vi "final.vi"() -> ()   [LabVIEW 2022 SP3]
uses:
  <vilib>/Utility/miscctls.llb/LVRectTypeDef.ctl
panel:
  in  "3 4":bool
  out "Time/Date":string
  in  "3 3":bool
  in  "3 2":bool
  in  "3":bool
  in  "2":bool
  in  "1":bool
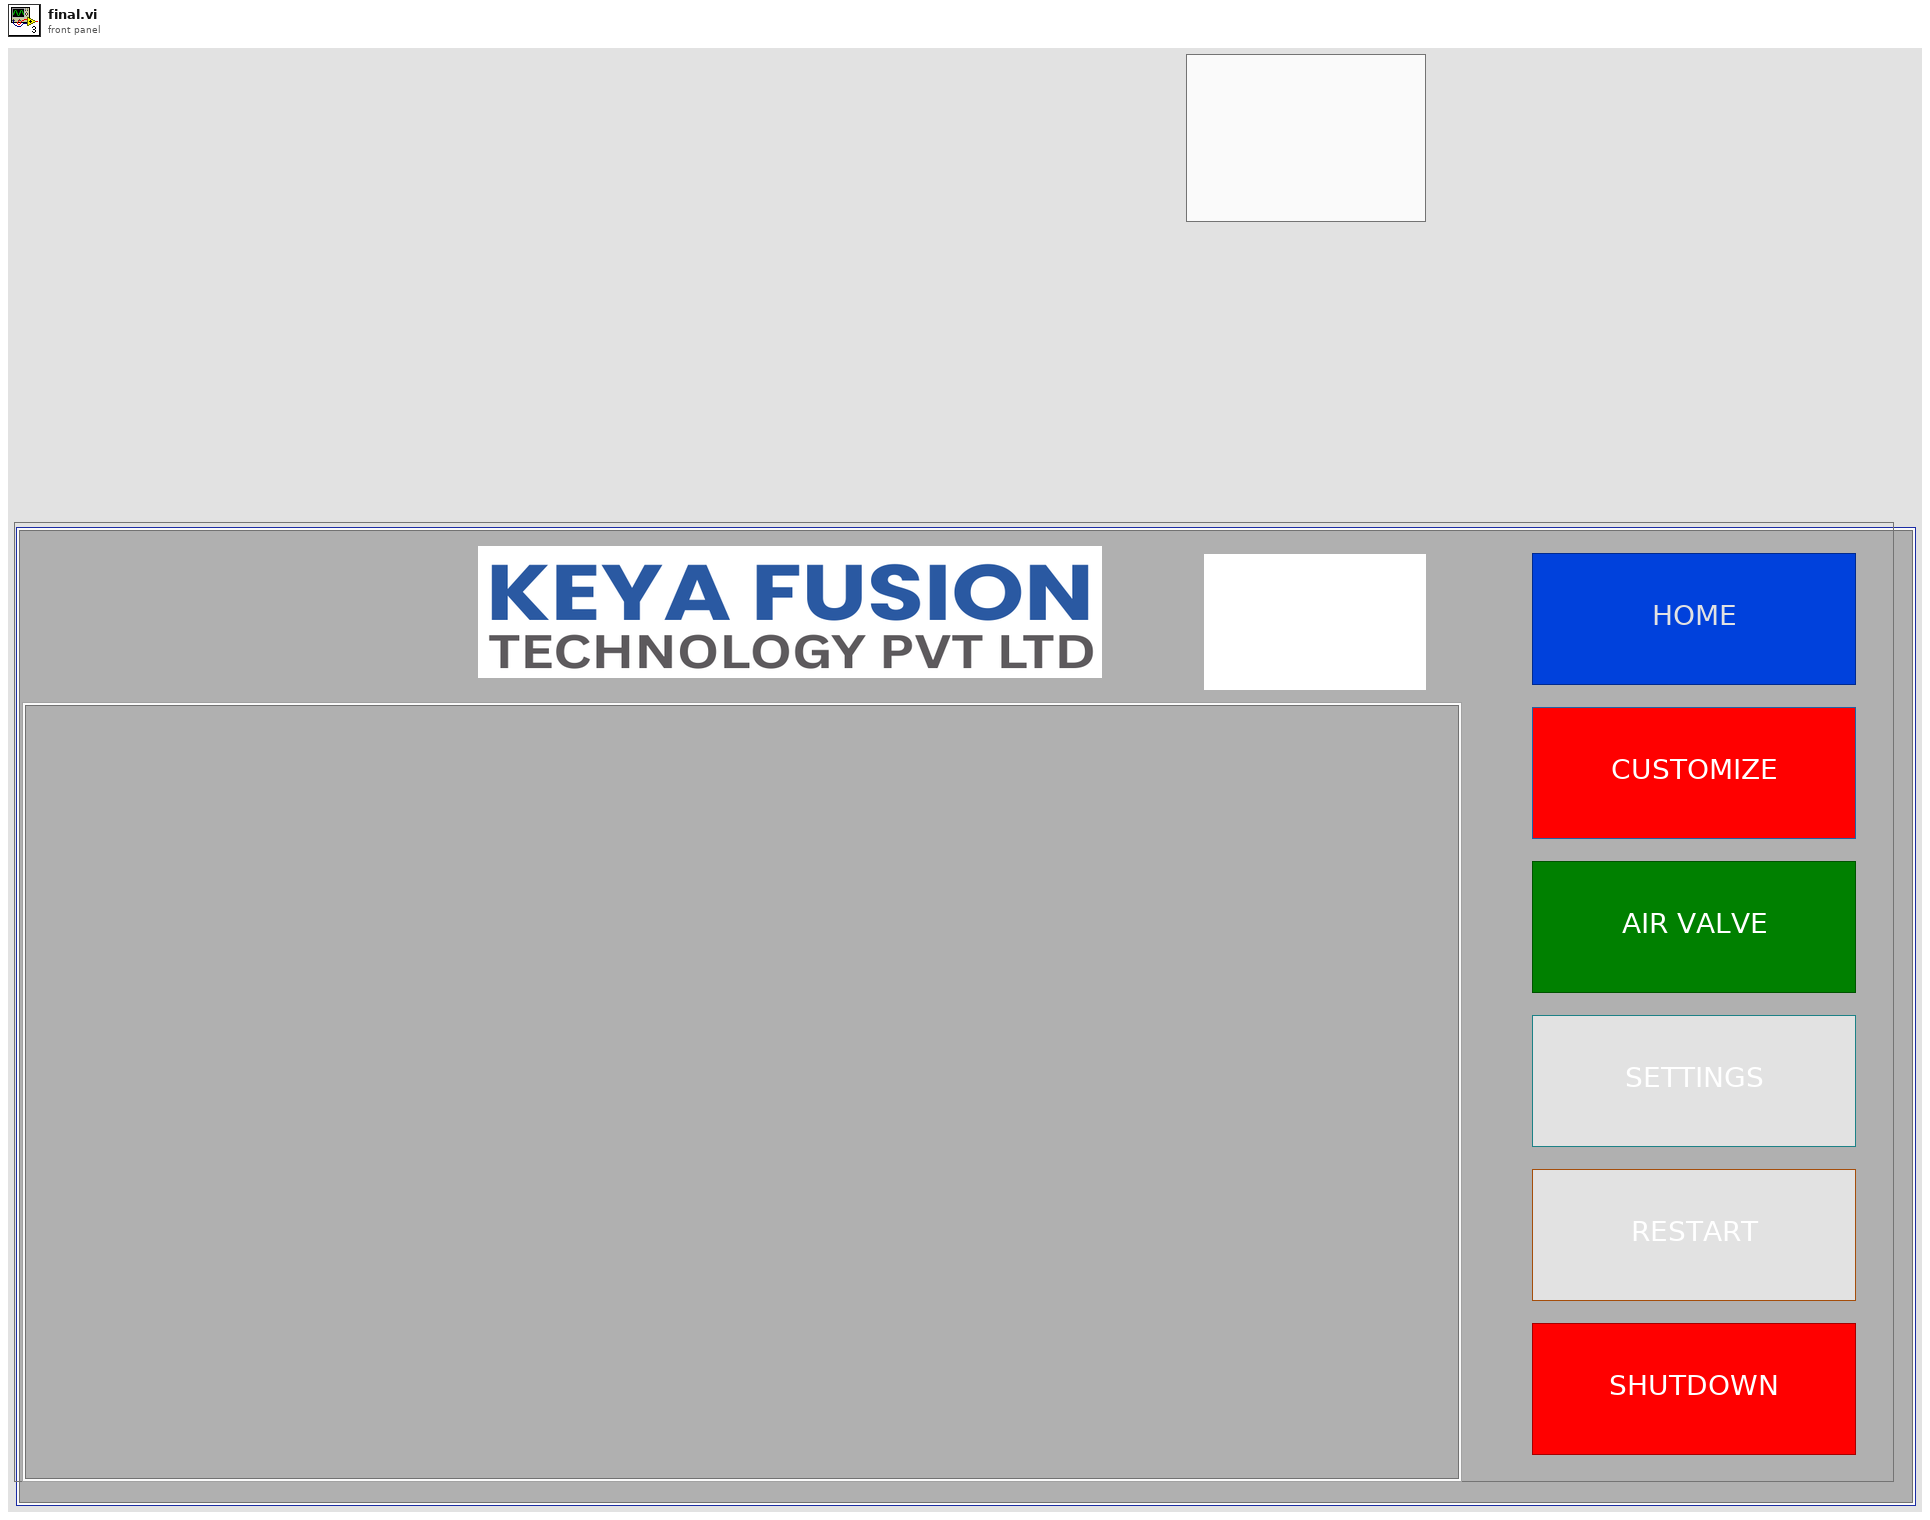
[diagram p1: front panel]
types:
  T1 = typedef "LVRectTypeDef.ctl" = cluster{"Left":i16, "Top":i16, "Right":i16, "Bottom":i16}
  T2 = typedef "LVDateTimeRec.ctl" = cluster{"fractional second":dbl, "second":i32, "minute":i32, "hour":i32, "day of month":i32, "month":i32, "year":i32, "day of week":i32, "day of year":i32, "DST":i32}
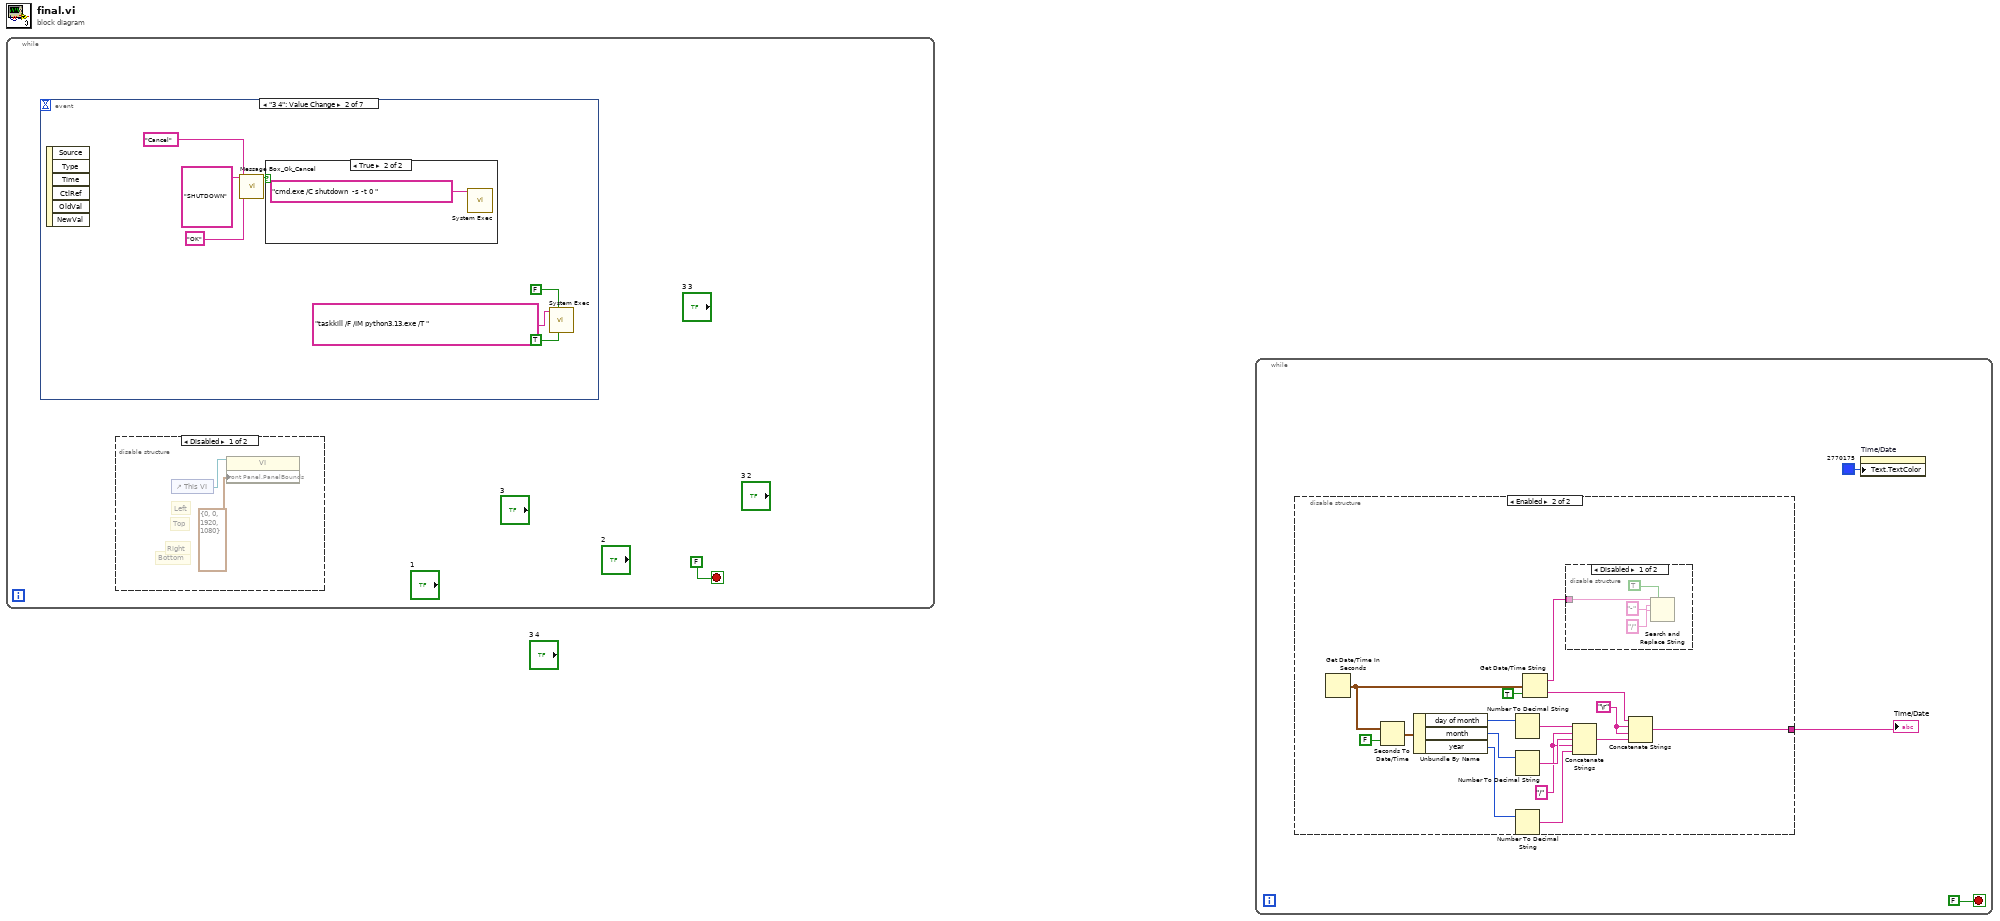
[diagram p0: block diagram]
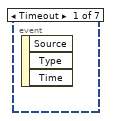
[diagram p5: hidden frame]
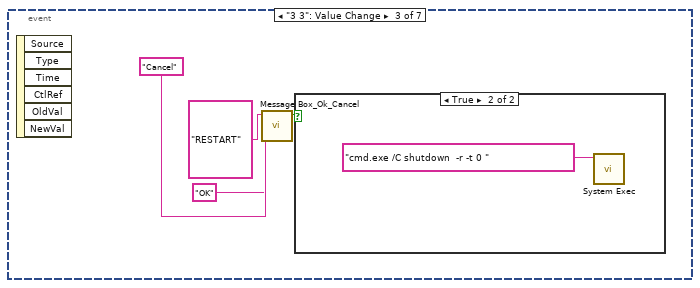
[diagram p7: hidden frame]
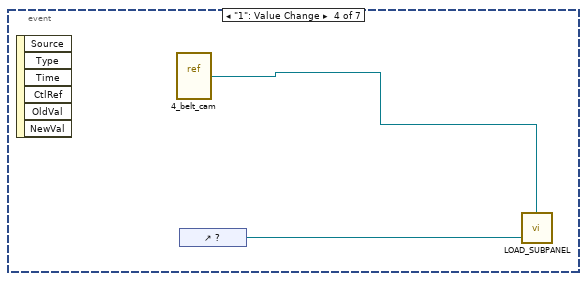
[diagram p9: hidden frame]
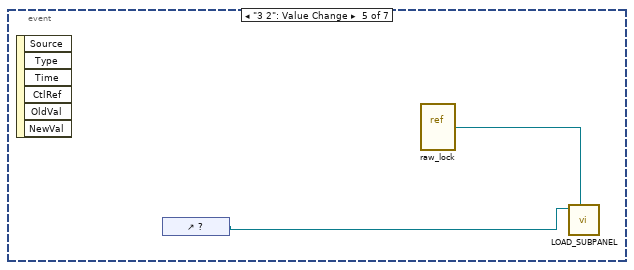
[diagram p10: hidden frame]
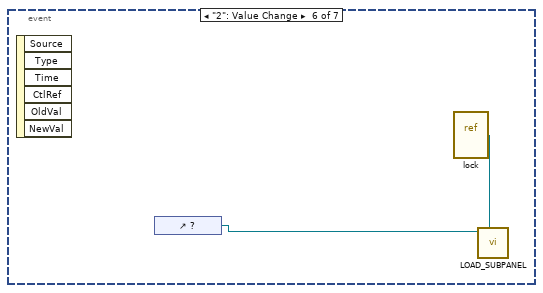
[diagram p11: hidden frame]
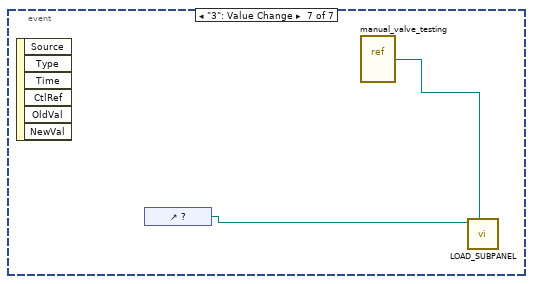
[diagram p12: hidden frame]
diagram:
  n1 = while {
    stop <- FALSE stop-if-true
    n2 = event shown="[1] \"3 4\": Value Change" {
      selector: _ -> [_ _ _ _ _ _ _]
      dyn-events: _ -> [_ _ _ _ _ _ _]
      timeout: _ -> [_ _ _ _ _ _ _]
      event Timeout {
        n3 = event-data() -> ()  [unwired: 1 in, 3 out]
      }
      event "3 4": Value Change {
        n4 = event-data() -> ()  [unwired: 1 in, 6 out]
        n5 = call "Message Box_Ok_Cancel.vi"("Cancel_buttonName"="Cancel", "Ok_buttonName"="OK", "Message"="SHUTDOWN") -> ("True/False"=w4:bool)  [unwired: 8 in]
        n6 = case shown="True" w4 {
          frame False {
          }
          frame True {
            n7 = call <vilib>:"System Exec.vi"("command line"="cmd.exe /C shutdown  -s -t 0 ") -> ()  [unwired: 7 in, 4 out]
          }
        }
        n8 = call <vilib>:"System Exec.vi"("run minimized? (F)"=TRUE, "wait until completion? (T)"=FALSE, "command line"="taskkill /F /IM python3.13.exe /T ") -> ()  [unwired: 5 in, 4 out]
      }
      event "3 3": Value Change {
        n9 = event-data() -> ()  [unwired: 1 in, 6 out]
        n10 = call "Message Box_Ok_Cancel.vi"("Cancel_buttonName"="Cancel", "Ok_buttonName"="OK", "Message"="RESTART") -> ("True/False"=w15:bool)  [unwired: 8 in]
        n11 = case shown="True" w15 {
          frame False {
          }
          frame True {
            n12 = call <vilib>:"System Exec.vi"("command line"="cmd.exe /C shutdown  -r -t 0 ") -> ()  [unwired: 7 in, 4 out]
          }
        }
      }
      event "1": Value Change {
        n13 = event-data() -> ()  [unwired: 1 in, 6 out]
        n14 = vi-ref "4_belt_cam.vi"() -> (w17:refnum<vi>)
        n15 = control-ref of="?"() -> (w18:refnum<vi>)
        n16 = call "LOAD_SUBPANEL.vi"("SubPanel in"=w18, "VI Ref"=w17) -> ()  [unwired: 8 in, 1 out]
      }
      event "3 2": Value Change {
        n17 = event-data() -> ()  [unwired: 1 in, 6 out]
        n18 = control-ref of="?"() -> (w19:refnum<vi>)
        n19 = vi-ref "raw_lock.vi"() -> (w20:refnum<vi>)
        n20 = call "LOAD_SUBPANEL.vi"("SubPanel in"=w19, "VI Ref"=w20) -> ()  [unwired: 8 in, 1 out]
      }
      event "2": Value Change {
        n21 = event-data() -> ()  [unwired: 1 in, 6 out]
        n22 = control-ref of="?"() -> (w22:refnum<vi>)
        n23 = vi-ref "lock.vi"() -> (w21:refnum<vi>)
        n24 = call "LOAD_SUBPANEL.vi"("SubPanel in"=w22, "VI Ref"=w21) -> ()  [unwired: 8 in, 1 out]
      }
      event "3": Value Change {
        n25 = event-data() -> ()  [unwired: 1 in, 6 out]
        n26 = control-ref of="?"() -> (w24:refnum<vi>)
        n27 = vi-ref "manual_valve_testing.vi"() -> (w23:refnum<vi>)
        n28 = call "LOAD_SUBPANEL.vi"("SubPanel in"=w24, "VI Ref"=w23) -> ()  [unwired: 8 in, 1 out]
      }
    }
    n29 = disable-structure shown="Disabled" {
      frame Disabled {
        # "Bottom"
        # "Right"
        # "Top"
        # "Left"
        n30 = control-ref of="This VI"() -> (w3:refnum<vi>)
        n31 = property class="VI"(reference=w3, "Front Panel.PanelBounds"=T1 {"Left"=0, "Top"=0, "Right"=1920, "Bottom"=1080} ("Front Panel Window:Panel Bounds")) -> ()  [unwired: 1 in, 2 out]
      }
      frame Enabled {
      }
    }
  }
  n32 = while {
    stop <- FALSE stop-if-true
    n33 = disable-structure shown="Enabled" {
      disable-tunnel: [_ w29] -> w27
      frame Disabled {
      }
      frame Enabled {
        w32 = "/" ("string")
        w31 = "\r"
        n34 = Get Date/Time In Seconds() -> (seconds since 1Jan1904=w43:timestamp)
        n35 = Seconds To Date/Time(time stamp (now)=w43, to UTC (F)=FALSE) -> (date time rec=w42:T2)
        n36 = Unbundle By Name(w42) -> ("day of month"=w36:i32, "month"=w37:i32, "year"=w38:i32)
        n37 = Number To Decimal String(number=w36) -> (decimal integer string=w39:string)  [unwired: 1 in]
        n38 = Number To Decimal String(number=w37) -> (decimal integer string=w40:string)  [unwired: 1 in]
        n39 = Number To Decimal String(number=w38) -> (decimal integer string=w41:string)  [unwired: 1 in]
        n40 = Get Date/Time String(seconds (now)=w43, want seconds? (F)=TRUE) -> (date string=w35:string, time string=w34:string)  [unwired: 1 in]
        n41 = disable-structure shown="Disabled" {
          disable-tunnel: w35 -> [w47 _]
          frame Disabled {
            n42 = Search and Replace String(replace all?=TRUE ("replace all? (F)"), input string=w47, search string="-", replace string="/" ("replace string (\"\")")) -> ()  [unwired: 4 in, 4 out]
          }
          frame Enabled {
          }
        }
        n43 = Concatenate Strings(w39, w32, w40, w32, w41) -> (w28:string)
        n44 = Concatenate Strings(w34, w31, w31, w28) -> (w29:string)
      }
    }
    "Time/Date" <- w27
    n45 = property on="Time/Date" class="Str"("Text.TextColor"=u32 2770175 ("Text.Text Colors:Text Color")) -> ()  [unwired: 2 in, 2 out]
  }
